vi "Utility Path Exist.vi"(11 "Path":path) -> (3 "Exists?":bool)   [LabVIEW 2020]
doc: "This VI checks if a file or folder exists. If it does exist, it will output a TRUE. Also, if the path is blank, the VI will output FALSE."
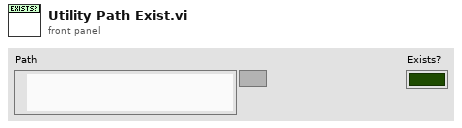
[diagram p1: front panel]
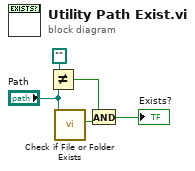
[diagram p0: block diagram]
diagram:
  n1 = Not Equal?(x=path "", y="Path") -> (x != y?=w3:bool)
  n2 = call <vilib>:"Check if File or Folder Exists.vi"("path"="Path") -> ("file or folder exists?"=w2:bool)  [unwired: 8 in, 2 out]
  n3 = And(x=w3, y=w2) -> (x .and. y?=→"Exists?":bool)
